vi "PC_SDSG to SDSM.vi"() -> ()   [LabVIEW 2021]
uses:
  Static Digital State Measurement/DAQ_Static Digital State Measurement.lvlib
  Static Digital State Generation/DAQ_Static Digital State Generation.lvlib
panel:
  out "Channel Identifiers Source":refnum<k21>[](array[refnum])=["Dev1/port0/line16", "Dev1/port0/line17", "Dev1/port1/line2", "Dev1/port1/line5"]
  out "Line States":bool[](array[boolean])=[TRUE, FALSE, TRUE, FALSE]
  out "Channel Line Identifiers Measurement":refnum<k21>[](array[refnum])=["Dev1/port0/line18", "Dev1/port0/line19", "Dev1/port1/line3", "Dev1/port1/line6"]
  out "error out":errorcluster
  in  "Data to Write":bool[](array[boolean])=[TRUE, FALSE, TRUE, FALSE]
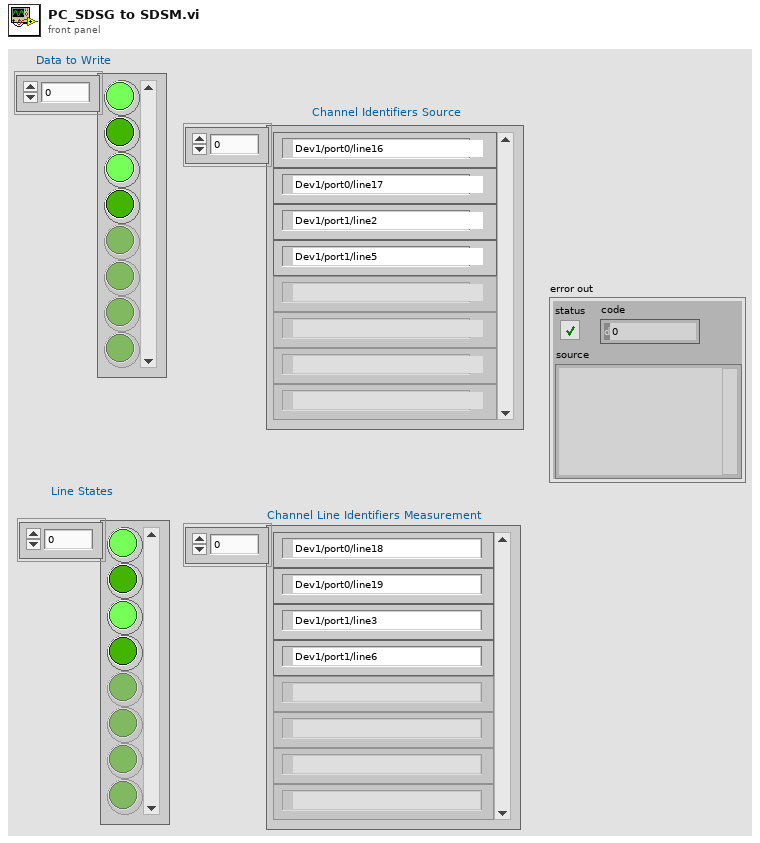
[diagram p1: front panel]
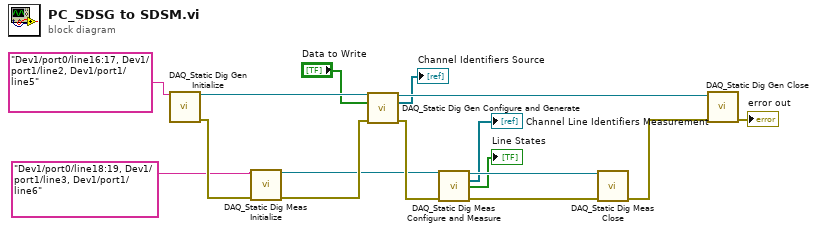
[diagram p0: block diagram]
diagram:
  n1 = call "DAQ_Static Dig Gen Initialize.vi"("Physical Channels"=tag "Dev1/port0/line16:17, Dev1/port1/line2, Dev1/port1/line5") -> ("DAQmx Task Out"=w16:refnum<k21>, "error out"=w14:errorcluster)  [unwired: 13 in]
  n2 = call "DAQ_Static Dig Meas Initialize.vi"("Physical Channels"=tag "Dev1/port0/line18:19, Dev1/port1/line3, Dev1/port1/line6", "error in"=w14) -> ("DAQmx Task Out"=w7:refnum<k21>, "error out"=w13:errorcluster)  [unwired: 12 in]
  n3 = call "DAQ_Static Dig Gen Configure and Generate.vi"("DAQmx Task In"=w16, "Data to Write"="Data to Write", "error in"=w13) -> ("DAQmx Task Out"=w15:refnum<k21>, "Channel Identifiers"=→"Channel Identifiers Source":refnum<k21>[], "error out"=w11:errorcluster)  [unwired: 10 in]
  n4 = call "DAQ_Static Dig Meas Configure and Measure.vi"("DAQmx Task In"=w7, "error in"=w11) -> ("DAQmx Task Out"=w6:refnum<k21>, "Channel Line Identifiers"=→"Channel Line Identifiers Measurement":refnum<k21>[], "Line States"=→"Line States":bool[], "error out"=w10:errorcluster)  [unwired: 10 in]
  n5 = call "DAQ_Static Dig Meas Close.vi"("DAQmx Task In"=w6, "error in"=w10) -> ("error out"=w9:errorcluster)  [unwired: 13 in]
  n6 = call "DAQ_Static Dig Gen Close.vi"("DAQmx Task In"=w15, "error in"=w9) -> ("error out"=→"error out":errorcluster)  [unwired: 13 in]
